vi "PH_PowerUnit_BaseClass.set Status.vi"(0 "VI in":refnum<vi>, 2 "Current PU Status":T1 items=["no info", "off/false/out", "on/true/in", "Failure", "Alarm", "Status 1", "Status 2", "Status 3"], 5 "error in (no error)":errorcluster) -> (14 "VI out":refnum<vi>, 19 "error out":errorcluster)   [LabVIEW 2014, in "PH_PowerUnit_BaseClass.lvlib"]
uses:
  PH_PowerUnit_BaseClass.lvlib
  PH_StatusHandler/PH_StatusHandler.lvlib
  PH_StatusHandler/PH_StatusHandler.Status.ctl
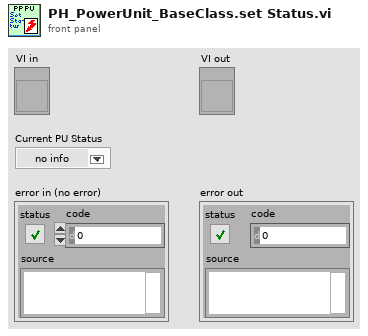
[diagram p1: front panel]
types:
  T1 = typedef "PH_StatusHandler.lvlib/PH_StatusHandler.Status.ctl" = i16
  T2 = typedef "PH_PowerUnit_BaseClass.lvlib/PH_PowerUnit_BaseClass.i attribute.ctl" = cluster{"Constructor finished":bool, "PU":cluster{"In use":bool, "Service ID in use":i32, "GUI Ref":refnum<vi>}, "Enabling":cluster{"State":T3, "GUI Ref":refnum<vi>}, "Timing":cluster{"Last Shot":dbl, "Time between Shots [Sec]":dbl, "Waiting Time over?":bool, "Service ID Waiting Time":i32, "GUI Ref":refnum<vi>, "Instance":cluster{"Status":T1, "linked?":bool, "GUI Ref":refnum<vi>}}, "Sequencer":cluster{"SM State":string, "GUI Ref":refnum<vi>, "linked":bool}, "Subscribed Trendmssgs":cluster{"Tagname":string, "Status":T1, "linked?":bool, "Shot Condition":T1, "GUI Ref":refnum<vi>}[], "PP PU":T4, "Default Voltage (V)":dbl, "GUI Refs":T5, "PSDB data":cluster{"Shot Voltage [V]":dbl, "State TO SM":T6, "Write 2 early":bool}, "State TO SM":T6}
  T3 = typedef "Enabling State.ctl" = i32
  T4 = typedef "PH_Common.PP PUs.ctl" = enum16{"no Info", "PA-19mm-1", "PA-19mm-2", "PA-45mm-PILC", "PA-45mm-MAIN", "MA-PU-1", "MA-PU-2", "MA-PU-3", "MA-PU-4", "MA-PU-5", "MA-PU-6", "MA-FR", "MA-PILC", "PA-45mm-DP"}
  T5 = typedef "PH_PowerUnit_BaseClass.lvlib/PH_PowerUnit_BaseClass.GUI Refs.ctl" = cluster{"Delete Inst":refnum<vi>, "State TO SM":refnum<vi>, "State SM":refnum<vi>, "Fire":refnum<vi>}
  T6 = typedef "PH_PowerUnit_BaseClass.lvlib/PH_PowerUnit_BaseClass.SM States.ctl" = enum16{".", "Stand by", "Switch PU on", "Configure", "Set Default Voltage", "Set STANDBY", "Set READY", "Wait for Shot Cmd", "Open Dump Rods", "Open Ross Relais", "Close Ross Relais", "Switch PSU on", "Switch PSU off", "Charge", "Switch GD Channel on", "Close Dump Rods", "Rods-TO", "RR-TO", "PSU-TO", "Trigger-TO"}
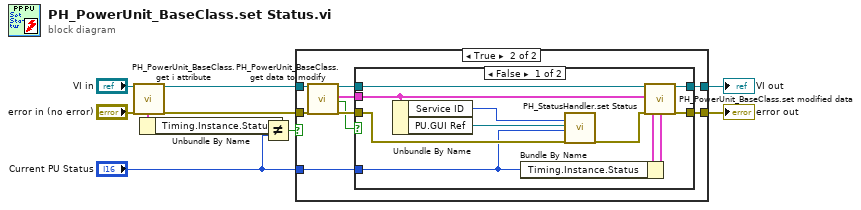
[diagram p0: block diagram]
diagram:
  n1 = call "PH_PowerUnit_BaseClass.get i attribute.vi"("i ref in"="VI in", "error in (no error)"="error in (no error)") -> ("i ref out"=w8:refnum<vi>, "i attribute"=w4:T2, "error out"=w6:errorcluster)  [unwired: 15 in]
  n2 = Unbundle By Name(w4) -> ("Timing.Instance.Status"=w10:T1)
  n3 = Not Equal?(x=w10, y="Current PU Status") -> (x != y?=w3:bool)
  n4 = case shown="True" w3 {
    tunnel: [w12 w20] -> w1
    tunnel: [w11 w19] -> w2
    tunnel: "Current PU Status" -> [_ w15]
    tunnel: w8 -> [w12 w14]
    tunnel: w6 -> [w11 w13]
    frame False {
    }
    frame True {
      n5 = call "PH_PowerUnit_BaseClass.get data to modify.vi"("i ref in"=w14, "error in (no error)"=w13) -> ("i ref out"=w21:refnum<vi>, "i attribute"=w18:T2, "timed out"=w16:bool, "error out"=w17:errorcluster)  [unwired: 14 in]
      n6 = case shown="False" w16 {
        tunnel: w21 -> [w31 w33]
        tunnel: [w26 w33] -> w20
        tunnel: [w25 w32] -> w19
        tunnel: w18 -> [w28 _]
        tunnel: w17 -> [w29 w32]
        tunnel: w15 -> [w24 _]
        frame False {
          n7 = Unbundle By Name(w28) -> ("Service ID"=w22:i32, "PU.GUI Ref"=w27:refnum<vi>)
          n8 = Bundle By Name(cluster=w28, "Timing.Instance.Status"=w24) -> (w30:T2)
          n9 = call "PH_StatusHandler.set Status.vi"("Service ID Status"=w22, "Ring in"=w27, "Status"=w24, "error in (no error)"=w29) -> ("error out"=w23:errorcluster)  [unwired: 15 in]
          n10 = call "PH_PowerUnit_BaseClass.set modified data.vi"("i ref in"=w31, "i attribute"=w30, "error in (no error)"=w23) -> ("i ref out"=w26:refnum<vi>, "error out"=w25:errorcluster)  [unwired: 15 in]
        }
        frame True {
        }
      }
    }
  }
  "error out" <- w2
  "VI out" <- w1
